vi "FT_Read_FT232-FT245R_EEPROM.vi"(0 "Handle":u32) -> (1 "FT_Status":u32(ring) items=["FT_OK", "FT_INVALID_HANDLE", "FT_DEVICE_NOT_FOUND", "FT_DEVICE_NOT_OPENED", "FT_IO_ERROR", "FT_INSUFFICIENT_RESOURCES", "FT_INVALID_PARAMETER", "FT_INVALID_BAUD_RATE", "FT_DEVICE_NOT_OPENED_FOR_ERASE", "FT_DEVICE_NOT_OPENED_FOR_WRITE", "FT_FAILED_TO_WRITE_DEVICE", "FT_EEPROM_READ_FAILED", "FT_EEPROM_WRITE_FAILED", "FT_EEPROM_ERASE_FAILED", "FT_EEPROM_NOT_PRESENT", "FT_EEPROM_NOT_PROGRAMMED", "FT_INVALID_ARGS", "FT_NOT_SUPPORTED", "FT_OTHER_ERROR"], 2 "FT232-FT245R EEPROM Contents":T1={"Vendor ID"=0, "Product ID"=0, "Manufacturer"="", "Manufacturer ID"="", "Description"="", "Serial Number"="", "Max Power (mA)"=0, "PnP"=0, "Self Powered"=0, "Remote Wake-Up"=0, "Use Ext Osc"=0, "High Drive IOs"=0, "Endpoint Size"=64, "Pull Down Enable"=0, "Serial Number Enable"=0, "Invert TXD"=0, "Invert RXD"=0, "Invert RTS"=0, "Invert CTS"=0, "Invert DTR"=0, "Invert DSR"=0, "Invert DCD"=0, "Invert RI"=0, "CBus0"=0, "CBus1"=0, "CBus2"=0, "CBus3"=0, "CBus4"=0, "Is D2XX"=0} {"Is D2XX" items=["VCP", "D2XX"]; "CBus4" items=["TXDEN", "PWRON#", "TXLED#", "RXLED#", "TX & RXLED#", "SLEEP#", "48MHz Clock", "24MHz Clock", "12MHz Clock", "6MHz Clock"]; "CBus3" items=["TXDEN", "PWRON#", "TXLED#", "RXLED#", "TX & RXLED#", "SLEEP#", "48MHz Clock", "24MHz Clock", "12MHz Clock", "6MHz Clock", "IO Mode", "Bit-Bang WRn", "Bit-Bang RDn"]; "CBus2" items=["TXDEN", "PWRON#", "TXLED#", "RXLED#", "TX & RXLED#", "SLEEP#", "48MHz Clock", "24MHz Clock", "12MHz Clock", "6MHz Clock", "IO Mode", "Bit-Bang WRn", "Bit-Bang RDn"]; "CBus1" items=["TXDEN", "PWRON#", "TXLED#", "RXLED#", "TX & RXLED#", "SLEEP#", "48MHz Clock", "24MHz Clock", "12MHz Clock", "6MHz Clock", "IO Mode", "Bit-Bang WRn", "Bit-Bang RDn"]; "CBus0" items=["TXDEN", "PWRON#", "TXLED#", "RXLED#", "TX & RXLED#", "SLEEP#", "48MHz Clock", "24MHz Clock", "12MHz Clock", "6MHz Clock", "IO Mode", "Bit-Bang WRn", "Bit-Bang RDn"]; "Invert RI" items=["RI Not Inverted", "RI Inverted"]; "Invert DCD" items=["DCD Not Inverted", "DCD Inverted"]; "Invert DSR" items=["DSR Not Inverted", "DSR Inverted"]; "Invert DTR" items=["DTR Not Inverted", "DTR Inverted"]; "Invert CTS" items=["CTS Not Inverted", "CTS Inverted"]; "Invert RTS" items=["RTS Not Inverted", "RTS Inverted"]; "Invert RXD" items=["RXD Not Inverted", "RXD Inverted"]; "Invert TXD" items=["TXD Not Inverted", "TXD Inverted"]; "Serial Number Enable" items=["Disabled", "Enabled"]; "Pull Down Enable" items=["Disabled", "Enabled"]; "Endpoint Size" items=["64"=64, "32"=32, "16"=16, "8"=8, "4"=4]; "High Drive IOs" items=["Disabled", "Enabled"]; "Use Ext Osc" items=["Internal Oscillator", "External Oscillator"]; "Remote Wake-Up" items=["Disabled", "Enabled"]; "Self Powered" items=["Bus Powered", "Self Powered"]; "PnP" items=["Disabled", "Enabled"]; "Product ID" format="%x"; "Vendor ID" format="%x"})   [LabVIEW 2019, in "D2XX_Functions.lvlib"]
uses:
  D2XX_Functions.lvlib
  CDM v2.12.36.4 WHQL Certified/i386/ftd2xx.dll
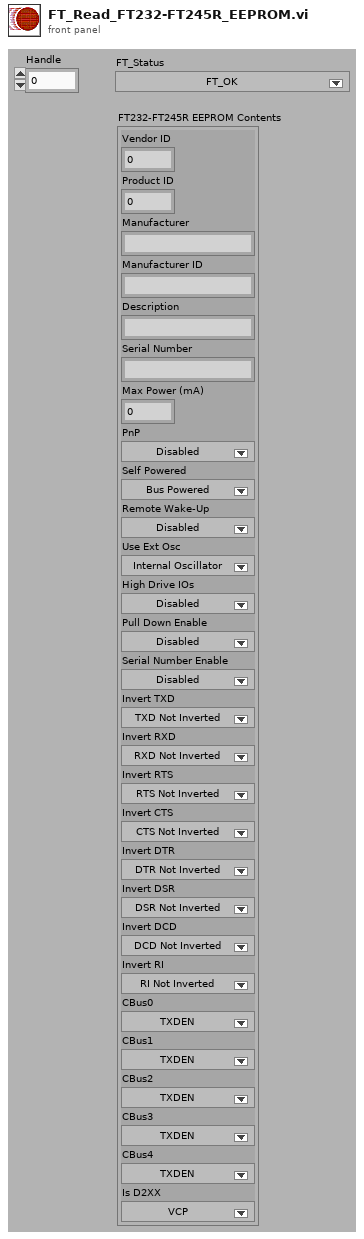
[diagram p1: front panel]
types:
  T1 = cluster{"Vendor ID":u16, "Product ID":u16, "Manufacturer":string, "Manufacturer ID":string, "Description":string, "Serial Number":string, "Max Power (mA)":u16, "PnP":u16, "Self Powered":u16, "Remote Wake-Up":u16, "Use Ext Osc":u8, "High Drive IOs":u8, "Endpoint Size":u8, "Pull Down Enable":u8, "Serial Number Enable":u8, "Invert TXD":u8, "Invert RXD":u8, "Invert RTS":u8, "Invert CTS":u8, "Invert DTR":u8, "Invert DSR":u8, "Invert DCD":u8, "Invert RI":u8, "CBus0":u8, "CBus1":u8, "CBus2":u8, "CBus3":u8, "CBus4":u8, "Is D2XX":u8}
  T2 = cluster{"Signature 1":u32, "Signature 2":u32, "Version":u32, "Vendor ID":u16, "Product ID":u16, "Manufacturer":u32, "Manufacturer ID":u32, "Description":u32, "Serial Number":u32, "Max Power (mA)":u16, "PnP":u16, "Self Powered":u16, "Remote Wake-Up":u16, "Rev4":u8, "Iso In":u8, "Iso Out":u8, "Pull Down Enable":u8, "Serial Number Enable":u8, "USB Version Enable":u8, "USB Version":u16, "Rev5":u8, "Iso In A":u8, "Iso In B":u8, "Iso Out A":u8, "Iso Out B":u8, "Pull Down Enable 5":u8, "Serial Number Enable 5":u8, "USB Version Enable 5":u8, "USB Version 5":u16, "A Is High Current":u8, "B Is High Current":u8, "A Is 245 FIFO":u8, "A Is CPU FIFO":u8, "A Is Fast Serial":u8, "A Is VCP":u8, "B Is 245 FIFO":u8, "B Is CPU FIFO":u8, "B Is Fast Serial":u8, "B Is VCP":u8, "Use Ext Osc":u8, "High Drive IOs":u8, "Endpoint Size":u8, "Pull Down Enable R":u8, "Serial Number Enable R":u8, "Invert TXD":u8, "Invert RXD":u8, "Invert RTS":u8, "Invert CTS":u8, "Invert DTR":u8, "Invert DSR":u8, "Invert DCD":u8, "Invert RI":u8, "CBus0":u8, "CBus1":u8, "CBus2":u8, "CBus3":u8, "CBus4":u8, "R Is VCP":u8, "Pull Down Enable 7":u8, "Serial Number Enable 7":u8, "AL Slow Slew":u8, "AL Schmitt Input":u8, "AL Drive Current":u8, "AH Slow Slew":u8, "AH Schmitt Input":u8, "AH Drive Current":u8, "BL Slow Slew":u8, "BL Schmitt Input":u8, "BL Drive Current":u8, "BH Slow Slew":u8, "BH Schmitt Input":u8, "BH Drive Current":u8, "A Is 245 FIFO 7":u8, "A Is CPU FIFO 7":u8, "A Is Fast Serial 7":u8, "A Is VCP 7":u8, "B Is 245 FIFO 7":u8, "B Is CPU FIFO 7":u8, "B Is Fast Serial 7":u8, "B Is VCP 7":u8, "PowerSaveEnable":u8, "Pull Down Enable 8":u8, "Serial Number Enable 8":u8, "A Slow Slew":u8, "A Schmitt Input":u8, "A Drive Current":u8, "B Slow Slew":u8, "B Schmitt Input":u8, "B Drive Current":u8, "C Slow Slew":u8, "C Schmitt Input":u8, "C Drive Current":u8, "D Slow Slew":u8, "D Schmitt Input":u8, "D Drive Current":u8, "A RI Is TXDEN":u8, "B RI Is TXDEN":u8, "C RI Is TXDEN":u8, "D RI Is TXDEN":u8, "A Is VCP 8":u8, "B Is VCP 8":u8, "C Is VCP 8":u8, "D Is VCP 8":u8}
  T3 = cluster{"Vendor ID":u16, "Product ID":u16, "Manufacturer":string, "Manufacturer ID":string, "Description":string, "Serial Number":string, "Max Power (mA)":u16, "PnP":u16, "Self Powered":u16, "Remote Wake-Up":u16, "Use Ext Osc":u8, "High Drive IOs":u8, "Endpoint Size":u8, "Pull Down Enable R":u8, "Serial Number Enable R":u8, "Invert TXD":u8, "Invert RXD":u8, "Invert RTS":u8, "Invert CTS":u8, "Invert DTR":u8, "Invert DSR":u8, "Invert DCD":u8, "Invert RI":u8, "CBus0":u8, "CBus1":u8, "CBus2":u8, "CBus3":u8, "CBus4":u8, "R Is VCP":u8}
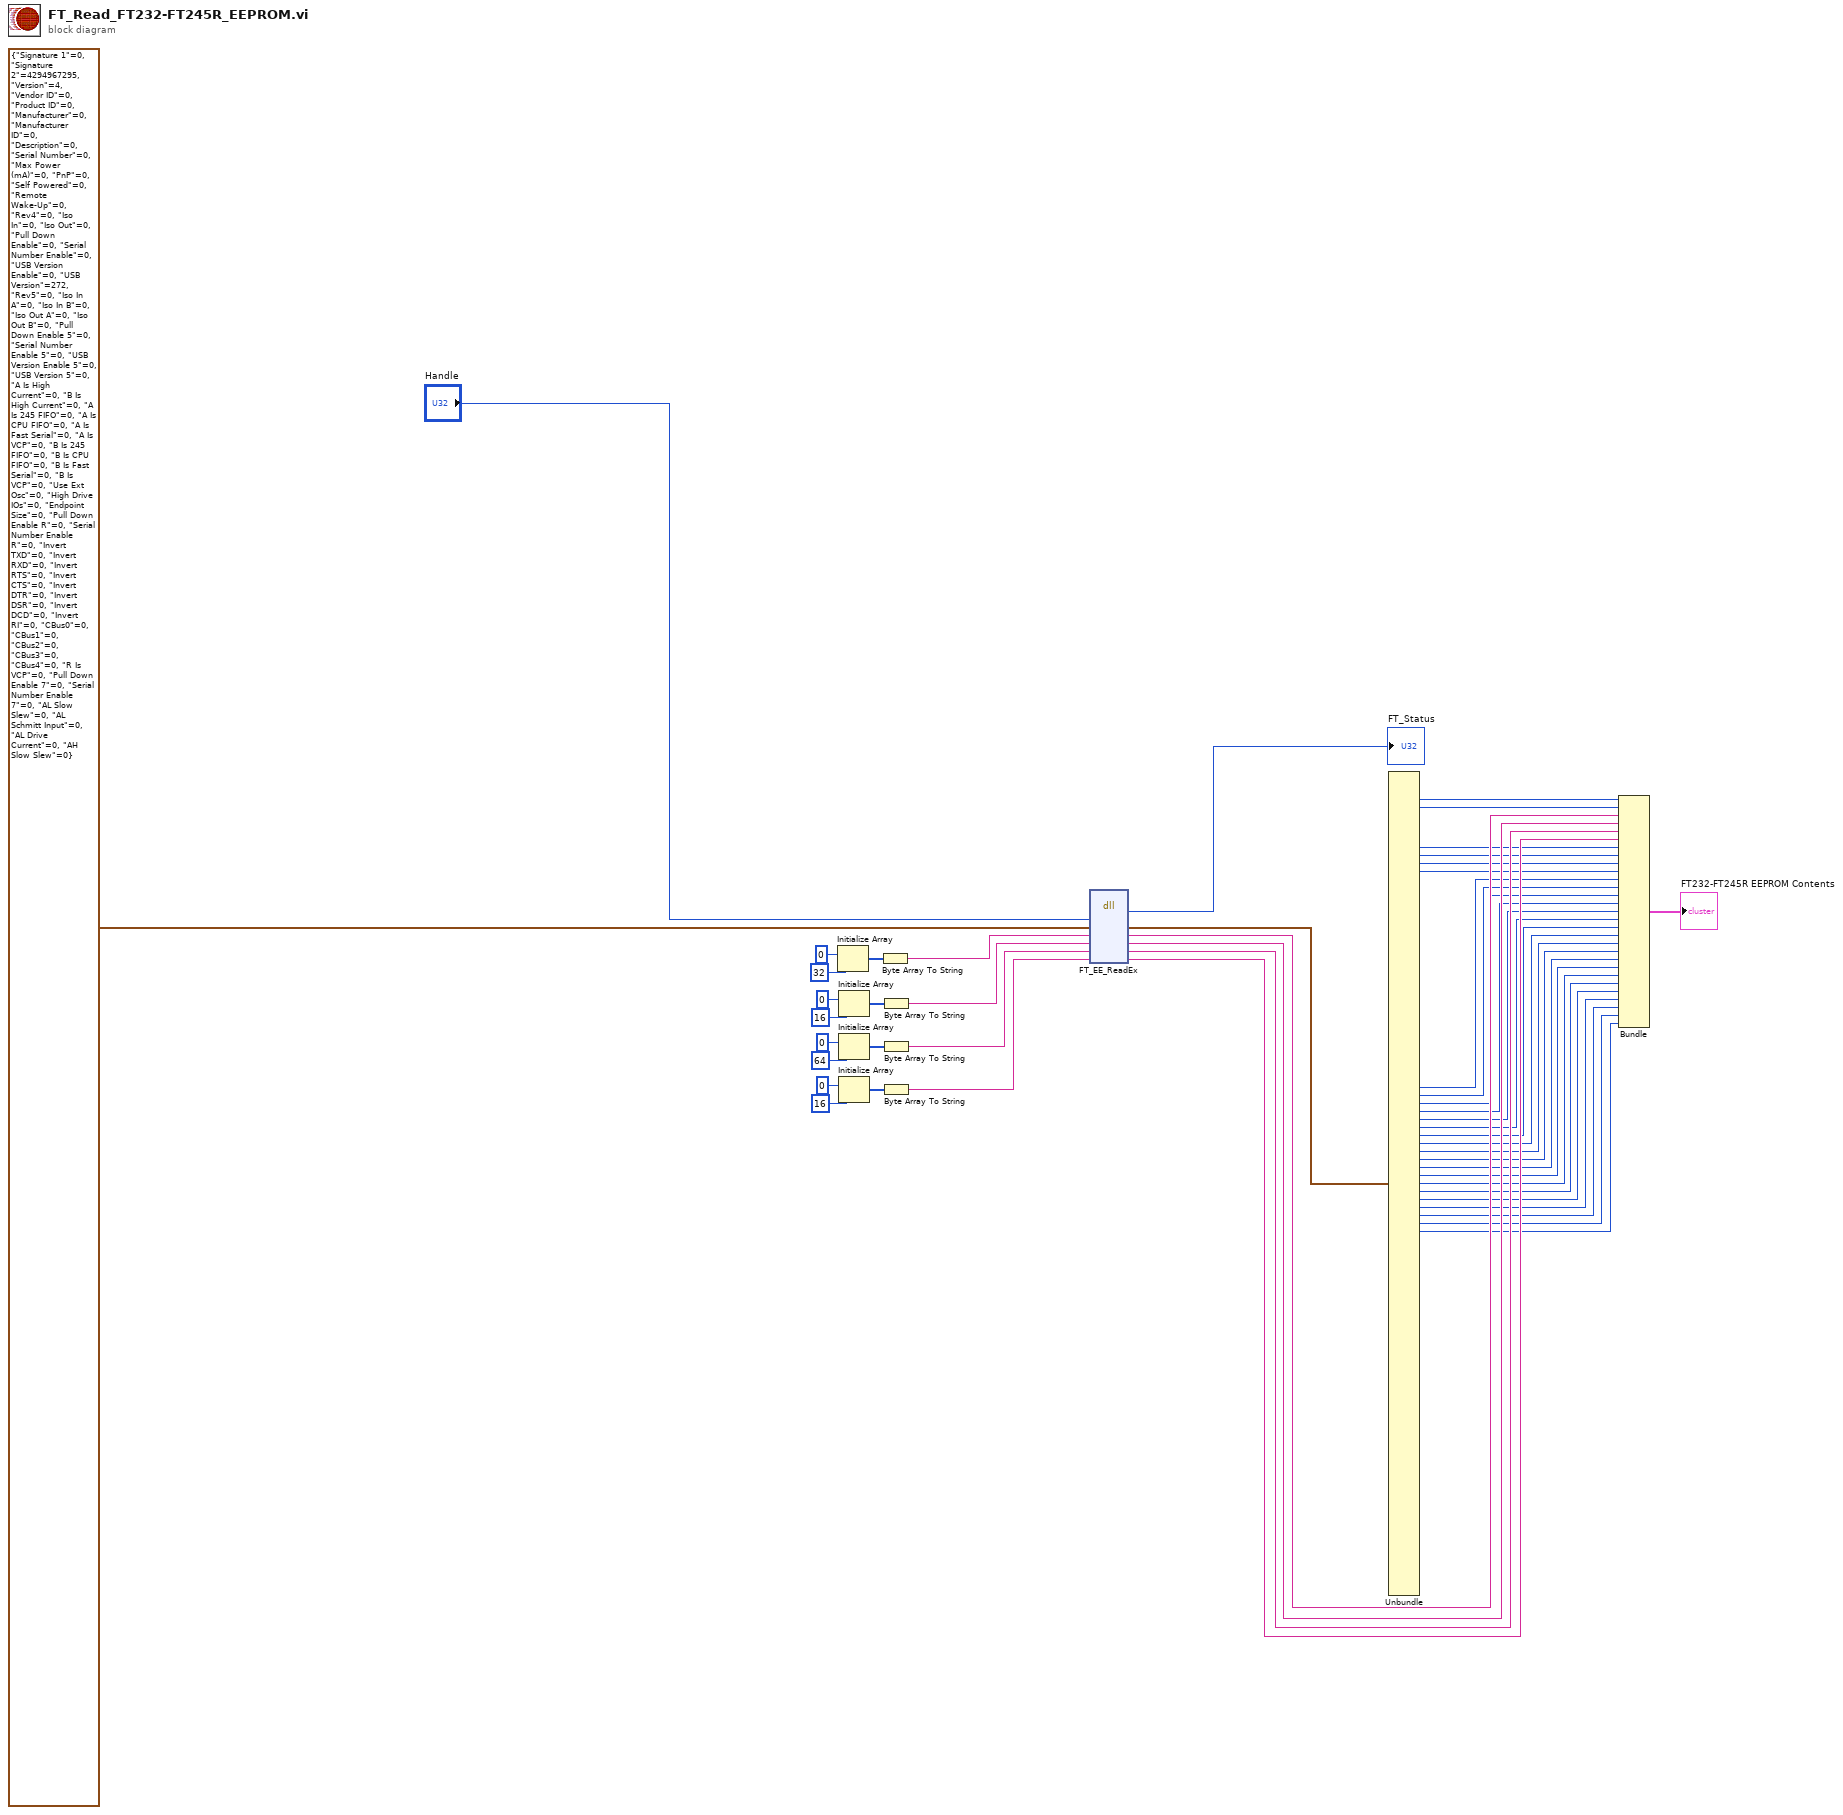
[diagram p0: block diagram]
diagram:
  n1 = Initialize Array(u8 0, 32 ("dimension size")) -> (w42:u8[])
  n2 = Initialize Array(u8 0, 16 ("dimension size")) -> (w40:u8[])
  n3 = Initialize Array(u8 0, 64 ("dimension size")) -> (w38:u8[])
  n4 = Initialize Array(u8 0, 16 ("dimension size")) -> (w36:u8[])
  n5 = Byte Array To String(unsigned byte array=w42) -> (string=w31:string)
  n6 = Byte Array To String(unsigned byte array=w40) -> (string=w30:string)
  n7 = Byte Array To String(unsigned byte array=w38) -> (string=w29:string)
  n8 = Byte Array To String(unsigned byte array=w36) -> (string=w28:string)
  n9 = dll-call lib="C:/Users/patrick/Documents/GitHub/Relay-Box/lvsrc/CDM v2.12.36.4 WHQL Certified/i386/FTD2XX.dll" fn="FT_EE_ReadEx"("Handle"="Handle", "FT232-FT245 EEPROM Contents 4"=T2 {"Signature 1"=0, "Signature 2"=4294967295, "Version"=4, "Vendor ID"=0, "Product ID"=0, "Manufacturer"=0, "Manufacturer ID"=0, "Description"=0, "Serial Number"=0, "Max Power (mA)"=0, "PnP"=0, "Self Powered"=0, "Remote Wake-Up"=0, "Rev4"=0, "Iso In"=0, "Iso Out"=0, "Pull Down Enable"=0, "Serial Number Enable"=0, "USB Version Enable"=0, "USB Version"=272, "Rev5"=0, "Iso In A"=0, "Iso In B"=0, "Iso Out A"=0, "Iso Out B"=0, "Pull Down Enable 5"=0, "Serial Number Enable 5"=0, "USB Version Enable 5"=0, "USB Version 5"=0, "A Is High Current"=0, "B Is High Current"=0, "A Is 245 FIFO"=0, "A Is CPU FIFO"=0, "A Is Fast Serial"=0, "A Is VCP"=0, "B Is 245 FIFO"=0, "B Is CPU FIFO"=0, "B Is Fast Serial"=0, "B Is VCP"=0, "Use Ext Osc"=0, "High Drive IOs"=0, "Endpoint Size"=0, "Pull Down Enable R"=0, "Serial Number Enable R"=0, "Invert TXD"=0, "Invert RXD"=0, "Invert RTS"=0, "Invert CTS"=0, "Invert DTR"=0, "Invert DSR"=0, "Invert DCD"=0, "Invert RI"=0, "CBus0"=0, "CBus1"=0, "CBus2"=0, "CBus3"=0, "CBus4"=0, "R Is VCP"=0, "Pull Down Enable 7"=0, "Serial Number Enable 7"=0, "AL Slow Slew"=0, "AL Schmitt Input"=0, "AL Drive Current"=0, "AH Slow Slew"=0, "AH Schmitt Input"=0, "AH Drive Current"=0, "BL Slow Slew"=0, "BL Schmitt Input"=0, "BL Drive Current"=0, "BH Slow Slew"=0, "BH Schmitt Input"=0, "BH Drive Current"=0, "A Is 245 FIFO 7"=0, "A Is CPU FIFO 7"=0, "A Is Fast Serial 7"=0, "A Is VCP 7"=0, "B Is 245 FIFO 7"=0, "B Is CPU FIFO 7"=0, "B Is Fast Serial 7"=0, "B Is VCP 7"=0, "PowerSaveEnable"=0, "Pull Down Enable 8"=0, "Serial Number Enable 8"=0, "A Slow Slew"=0, "A Schmitt Input"=0, "A Drive Current"=0, "B Slow Slew"=0, "B Schmitt Input"=0, "B Drive Current"=0, "C Slow Slew"=0, "C Schmitt Input"=0, "C Drive Current"=0, "D Slow Slew"=0, "D Schmitt Input"=0, "D Drive Current"=0, "A RI Is TXDEN"=0, "B RI Is TXDEN"=0, "C RI Is TXDEN"=0, "D RI Is TXDEN"=0, "A Is VCP 8"=0, "B Is VCP 8"=0, "C Is VCP 8"=0, "D Is VCP 8"=0}, "Manufacturer"=w31, "Manufacturer ID"=w30, "Description"=w29, "Serial Number"=w28) -> ("FT_Status"=→"FT_Status":u32, "FT232-FT245 EEPROM Contents 4"=w27:T2, "Manufacturer"=w46:string, "Manufacturer ID"=w48:string, "Description"=w47:string, "Serial Number"=w45:string)  [unwired: 4 in, 2 out]
  n10 = Unbundle(w27) -> ("Vendor ID"=w7:u16, "Product ID"=w6:u16, "Max Power (mA)"=w5:u16, "PnP"=w4:u16, "Self Powered"=w3:u16, "Remote Wake-Up"=w2:u16, "Use Ext Osc"=w26:u8, "High Drive IOs"=w25:u8, "Endpoint Size"=w24:u8, "Pull Down Enable R"=w23:u8, "Serial Number Enable R"=w22:u8, "Invert TXD"=w21:u8, "Invert RXD"=w20:u8, "Invert RTS"=w19:u8, "Invert CTS"=w18:u8, "Invert DTR"=w17:u8, "Invert DSR"=w16:u8, "Invert DCD"=w15:u8, "Invert RI"=w14:u8, "CBus0"=w13:u8, "CBus1"=w12:u8, "CBus2"=w11:u8, "CBus3"=w10:u8, "CBus4"=w9:u8, "R Is VCP"=w8:u8)  [unwired: 78 out]
  n11 = Bundle("Vendor ID"=w7, "Product ID"=w6, "Manufacturer"=w46, "Manufacturer ID"=w48, "Description"=w47, "Serial Number"=w45, "Max Power (mA)"=w5, "PnP"=w4, "Self Powered"=w3, "Remote Wake-Up"=w2, "Use Ext Osc"=w26, "High Drive IOs"=w25, "Endpoint Size"=w24, "Pull Down Enable R"=w23, "Serial Number Enable R"=w22, "Invert TXD"=w21, "Invert RXD"=w20, "Invert RTS"=w19, "Invert CTS"=w18, "Invert DTR"=w17, "Invert DSR"=w16, "Invert DCD"=w15, "Invert RI"=w14, "CBus0"=w13, "CBus1"=w12, "CBus2"=w11, "CBus3"=w10, "CBus4"=w9, "R Is VCP"=w8) -> (→"FT232-FT245R EEPROM Contents":T3)  [unwired: 1 in]
